vi "endsavedata.vi"(2 "错误输入":errorcluster, 3 "文件路径（使用对话框）":path, 4 "文本":string) -> (0 "错误输出":errorcluster, 1 "路径 2":path)   [LabVIEW 2020]
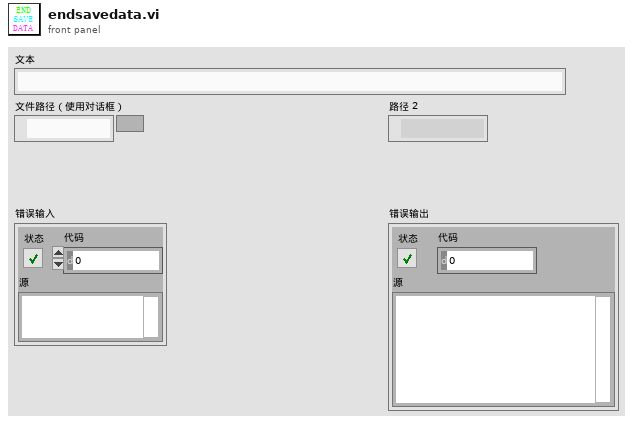
[diagram p1: front panel]
types:
  T1 = enum16{"open", "replace", "create", "open or create", "replace or create", "replace or create with confirmation"}
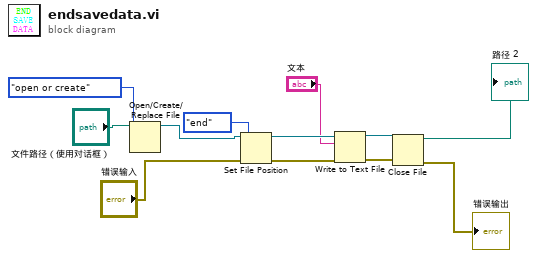
[diagram p0: block diagram]
diagram:
  n1 = Open/Create/Replace File(file path (use dialog)="文件路径（使用对话框）", operation (0:open)=T1."open or create" ("操作(0:open)")) -> (refnum out=w3:refnum<file>)  [unwired: 4 in, 2 out]
  n2 = Set File Position(refnum=w3, from (0:start)=enum16{"start", "end", "current"}."end" ("自（0:起始）"), error in="错误输入") -> (refnum out=w9:refnum<file>, error out=w8:errorcluster)  [unwired: 1 in]
  n3 = Write to Text File(file (use dialog)=w9, text="文本", error in=w8) -> (refnum out=w12:refnum<file>, error out=w11:errorcluster)  [unwired: 1 in, 1 out]
  n4 = Close File(refnum=w12, error in=w11) -> (path=→"路径 2":path, error out=→"错误输出":errorcluster)
